vi "test udp++2.vi"() -> ()   [LabVIEW 2017]
uses:
  UDP++.lvlib
panel:
  in  "stop":bool
  out "sumcheck":dbl[](array[numeric])
  out "Validation send":dbl[](array[numeric])
  in  "Numeric":i32=1000
  out "Array":dbl[](array[numeric])
  out "接收控制指令":dbl[](array[numeric])
  out "wifi_KongZ":bool
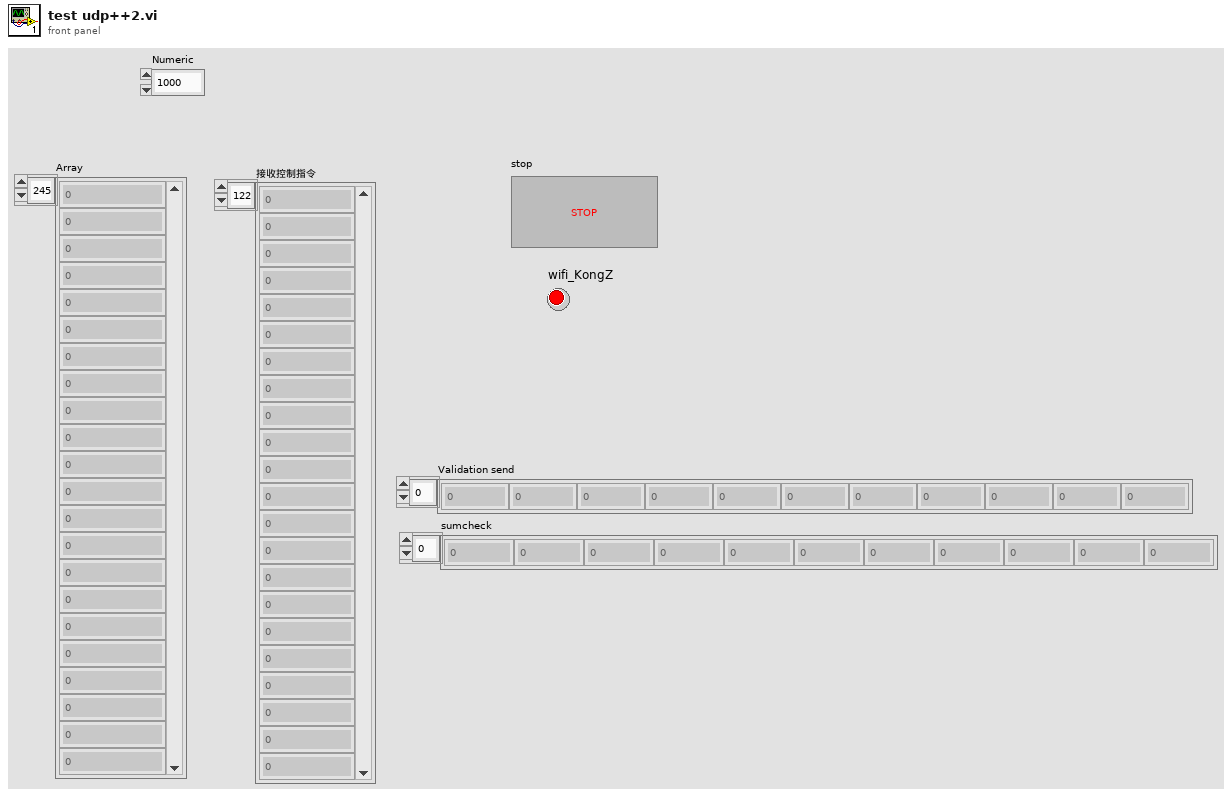
[diagram p1: front panel]
types:
  T1 = cluster{"本地IP":string, "本地端口":u16, "远程IP":string, "远程端口":u16}
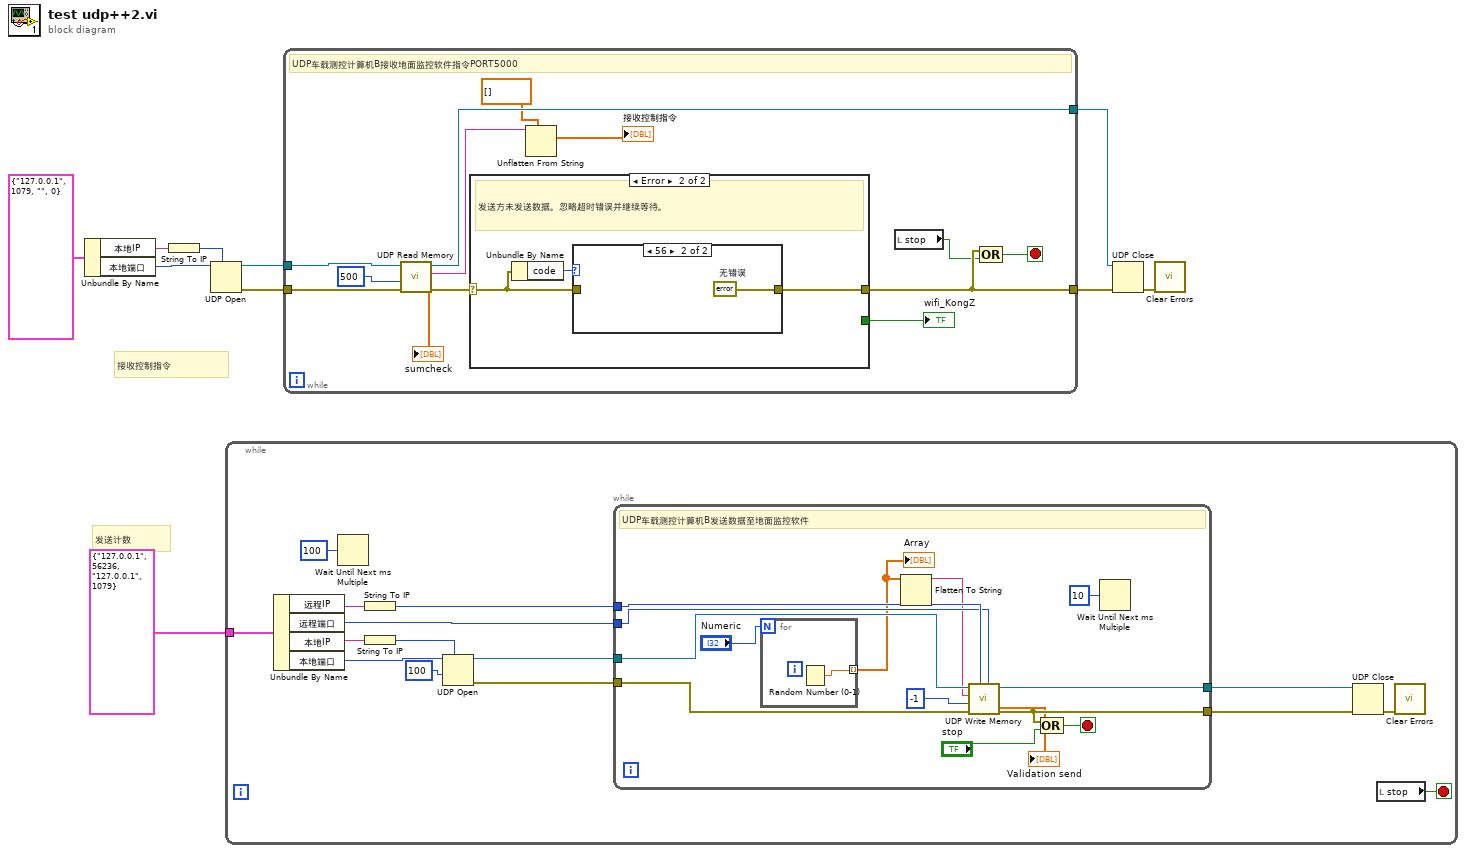
[diagram p0: block diagram]
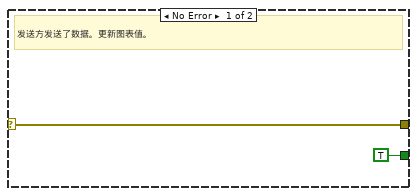
[diagram p2: hidden frame]
diagram:
  # "发送计数"
  # "接收控制指令"
  n1 = Unbundle By Name(T1 {"本地IP"="127.0.0.1", "本地端口"=1079, "远程IP"="", "远程端口"=0} ("UDP配置")) -> ("本地IP"=w3:string, "本地端口"=w2:u16)
  n2 = String To IP(1:w3) -> (0:w10:u32)
  n3 = UDP Open(7:w10, 11:w2) -> (port=w9:refnum<k16>, 0:w8:errorcluster)  [unwired: 3 in, 1 out]
  n4 = while {
    tunnel: T1 {"本地IP"="127.0.0.1", "本地端口"=56236, "远程IP"="127.0.0.1", "远程端口"=1079} ("UDP配置") -> [w16]
    stop <- w11 stop-if-true
    n5 = Unbundle By Name(w16) -> ("远程IP"=w13:string, "远程端口"=w12:u16, "本地IP"=w14:string, "本地端口"=w15:u16)
    n6 = Wait Until Next ms Multiple(millisecond multiple=u32 100 ("毫秒倍数")) -> ()  [unwired: 1 out]
    n7 = String To IP(1:w13) -> (0:w21:u32)
    n8 = String To IP(1:w14) -> (0:w23:u32)
    n9 = UDP Open(7:w23, 9:100 ("超时毫秒(25000)"), 11:w15) -> (port=w25:refnum<k16>, 0:w24:errorcluster)  [unwired: 2 in, 1 out]
    n10 = while {
      tunnel: [w36] -> w19
      tunnel: w25 -> [w39]
      tunnel: w24 -> [w37]
      tunnel: [w38] -> w18
      tunnel: w12 -> [w32]
      tunnel: w21 -> [w33]
      stop <- w35 stop-if-true
      # "UDP车载测控计算机B发送数据至地面监控软件"
      n11 = for {
        N: "Numeric" -> [_]
        tunnel: [w40] -> w30 mode=indexing
        n12 = Random Number (0-1)() -> (number: 0 to 1=w40:dbl)
      }
      "Array" <- w30
      n13 = Flatten To String(anything=w30) -> (data string=w29:string)  [unwired: 3 in, 2 out]
      n14 = call "UDP Write Memory.vi"("port or service name"=w32, "address"=w33, "error in (no error)"=w37, "超时毫秒(25000)"=-1, "String"=w29, "UDP Network Connection in"=w39) -> ("error out"=w36:errorcluster, "UDP Network Connection out"=w38:refnum<k16>, "checksum"=→"Validation send":dbl[])  [unwired: 3 in]
      n15 = Compound Arithmetic op=OR ("复合运算")(w36, "stop") -> (w35:bool)
      n16 = Wait Until Next ms Multiple(millisecond multiple=u32 10 ("毫秒倍数")) -> ()  [unwired: 1 out]
    }
    n17 = UDP Close(connection ID=w18, 8:w19) -> (error out=w17:errorcluster)  [unwired: 1 out]
    n18 = local read "stop"() -> (w11:bool)
    n19 = call <vilib>:"Clear Errors.vi"("error in (no error)"=w17) -> ()  [unwired: 5 in, 2 out]
  }
  n20 = while {
    tunnel: w9 -> [w53]
    tunnel: [w51] -> w6
    tunnel: w8 -> [w52]
    tunnel: [w50] -> w7
    stop <- w49 stop-if-true
    # "UDP车载测控计算机B接收地面监控软件指令PORT5000"
    n21 = call "UDP Read Memory.vi"("error in (no error)"=w52, "超时毫秒(25000)"=500, "UDP Network Connection in"=w53) -> ("error out"=w47:errorcluster, "String"=w45:string, "UDP Network Connection out"=w51:refnum<k16>, "checksum"=→"sumcheck":dbl[])  [unwired: 5 in]
    n22 = case shown="Error" w47 {
      selector: w47 -> [w55 w57]
      tunnel: [w55 w56] -> w50
      tunnel: [TRUE ("wifi_KongZ") _] -> w48
      frame No Error {
        # "发送方发送了数据。更新图表值。"
      }
      frame Error {
        # "发送方未发送数据。忽略超时错误并继续等待。"
        n23 = Unbundle By Name(w57) -> ("code"=w58:i32)
        n24 = case shown="56" w58 {
          tunnel: w57 -> [w59 _]
          tunnel: [w59 w60] -> w56
          frame Default {
          }
          frame 56 {
            w60 = errorcluster {"status"=FALSE, "code"=0, "source"=""}  # 无错误
          }
        }
      }
    }
    "wifi_KongZ" <- w48
    n25 = Unflatten From String(type=dbl[] [] ("接收控制指令"), binary string=w45) -> (value=→"接收控制指令":dbl[])  [unwired: 3 in, 2 out]
    n26 = local read "stop"() -> (w41:bool)
    n27 = Compound Arithmetic op=OR ("复合运算")(w50, w41) -> (w49:bool)
  }
  n28 = UDP Close(connection ID=w6, 8:w7) -> (error out=w5:errorcluster)  [unwired: 1 out]
  n29 = call <vilib>:"Clear Errors.vi"("error in (no error)"=w5) -> ()  [unwired: 5 in, 2 out]
